vi "Out of Bounds Exception.vi"(8 "error in (no error)":errorcluster, 11 "EPU452 in":refnum<class "EPU452.lvclass">) -> (0 "error out":errorcluster, 3 "EPU452 out":refnum<class "EPU452.lvclass">)   [LabVIEW 2018, in "EPU452.lvclass"]
uses:
  EPU452.lvclass
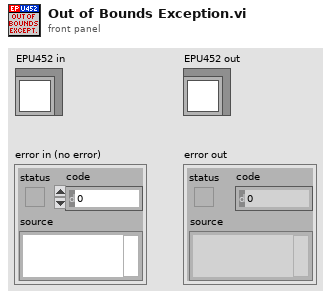
[diagram p1: front panel]
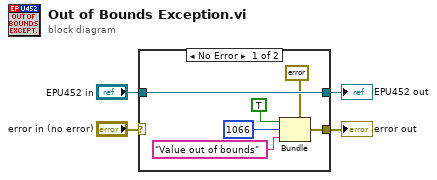
[diagram p0: block diagram]
diagram:
  n1 = case shown="No Error" "error in (no error)" {
    selector: "error in (no error)" -> [_ w12]
    tunnel: [w8 w12] -> w3
    tunnel: [w10 w11] -> w1
    tunnel: "EPU452 in" -> [w10 w11]
    frame No Error {
      n2 = Bundle(cluster=errorcluster {"status"=FALSE, "code"=0, "source"=""} ("error constant"), "status"=TRUE ("show call chain? (False)"), "code"=1066 ("error code (0)"), "source"="Value out of bounds" ("error message (\"\")")) -> (w8:errorcluster)
    }
    frame Error {
    }
  }
  "error out" <- w3
  "EPU452 out" <- w1
